vi "Handle Last Ack Core.vi"(4 "error in":errorcluster, 6 "Last Ack":refnum<class "Last Ack.lvclass">, 7 "Host MSS Test Actor in":refnum<class "Host MSS Test Actor.lvclass">) -> (0 "error out":errorcluster, 3 "Host MSS Test Actor out":refnum<class "Host MSS Test Actor.lvclass">)   [LabVIEW 2023, in "Host MSS Test Actor.lvlib" / "Host MSS Test Actor.lvclass"]
doc: "(<B>Filename</B>: Actor Framework.lvlib:Actor.lvclass:Handle Last Ack Core.vi)\n\nDefines how the caller actor responds to the Last Ack message from a nested actor. The Last Ack message is the final message a nested actor sends to its caller before it shuts down. The message contains information about the final state of the nested actor.\n\nBy default, this method does nothing except return any error the nested actor sent. A descendant class may override this method to define behavior."
uses:
  Host MSS Test Actor.lvclass
  <vilib>/ActorFramework/LastAck/Last Ack.lvclass
  <vilib>/ActorFramework/LastAck/Last Ack.lvclass/Last Ack.ctl
  Host MSS Test Actor.lvclass/Host MSS Test Actor.ctl
  <vilib>/ActorFramework/Actor/Actor.lvclass
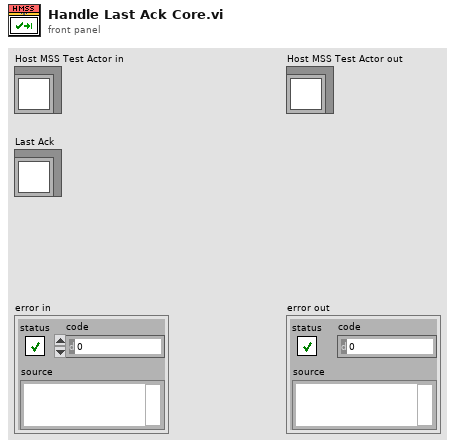
[diagram p1: front panel]
types:
  T1 = map{string, refnum<class "Message Enqueuer.lvclass">}
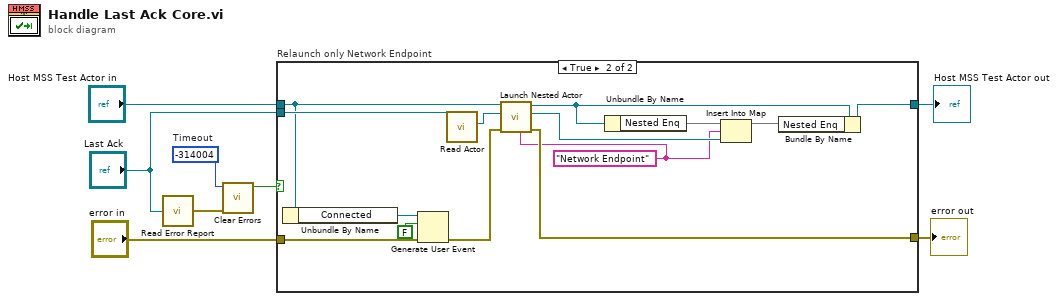
[diagram p0: block diagram]
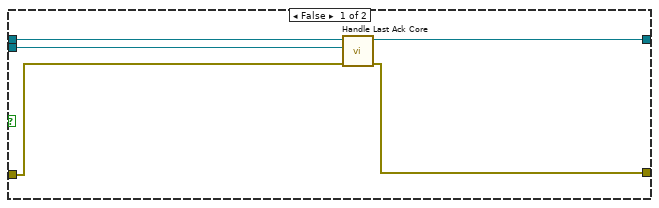
[diagram p2: hidden frame]
diagram:
  w7 = -314004  # Timeout
  n1 = call <vilib>:"Read Error Report.vi"("Last Ack"="Last Ack") -> ("error report"=w8:errorcluster)
  n2 = call <vilib>:"Clear Errors.vi"("error in (no error)"=w8, "specific error code to clear (0: all)"=w7) -> ("specific error cleared?"=w6:bool)  [unwired: 4 in, 1 out]
  n3 = case "Relaunch only Network Endpoint" shown="True" w6 {
    tunnel: "Host MSS Test Actor in" -> [w13 w16]
    tunnel: [w11 w27] -> w1
    tunnel: [w12 w23] -> w2
    tunnel: "Last Ack" -> [w10 w20]
    tunnel: "error in" -> [w9 w18]
    frame False {
      n4 = call-parent "Handle Last Ack Core.vi"("error in (no error)"=w9, "Last Ack"=w10, "Actor in"=w13) -> ("error out"=w11:errorcluster, "Actor out"=w12:refnum<class "Host MSS Test Actor.lvclass">)  [unwired: 3 in]
    }
    frame True {
      w21 = "Network Endpoint" ("key")
      n5 = Unbundle By Name(w16) -> ("Connected"=w15:refnum<user-event>)
      n6 = Generate User Event(user event=w15, event data cluster=FALSE ("event data"), error in=w18) -> (error out=w17:errorcluster)  [unwired: 1 in, 1 out]
      n7 = call <vilib>:"Read Actor.vi"("Last Ack"=w20) -> ("Actor"=w19:refnum<class "Actor.lvclass">)  [unwired: 10 in]
      n8 = call <vilib>:"Launch Nested Actor.vi"("Debug Alias"=w21, "error in (no error)"=w17, "Nested Actor"=w19, "Caller Actor in"=w16) -> ("error out"=w27:errorcluster, "Nested Actor's Enqueuer"=w24:refnum<class "Message Enqueuer.lvclass">, "Caller Actor out"=w26:refnum<class "Host MSS Test Actor.lvclass">)  [unwired: 5 in]
      n9 = Unbundle By Name(w26) -> ("Nested Enq"=w25:T1)
      n10 = Insert Into Map(map in=w25, key=w21, value=w24) -> (map out=w22:T1)  [unwired: 2 out]
      n11 = Bundle By Name(cluster=w26, "Nested Enq"=w22) -> (w23:refnum<class "Host MSS Test Actor.lvclass">)
    }
  }
  "Host MSS Test Actor out" <- w2
  "error out" <- w1
